vi "Write Ramp Volt.vi"(8 "error in":errorcluster, 10 "Voltage_Ramp":dbl, 11 "89XX in":refnum<class "89XX.lvclass">) -> (0 "error out":errorcluster, 3 "89XX out":refnum<class "89XX.lvclass">)   [LabVIEW 2019, in "89XX.lvlib" / "89XX.lvclass"]
uses:
  Library/89XX.lvclass
  C:/Users/Public/Documents/Development/builds/Engine/Monitored Actor.lvlibp/Monitored Actor/Monitored Actor/Monitored Actor.lvclass
  builds/Engine/Monitored Actor.lvlibp/Monitored Actor/Monitored Actor/Read Actor Label.vi
  builds/Instruments/PowerSupply.lvlibp/Library/PowerSupply.lvclass
  <vilib>/ErrorRing/Error Ring.xnode
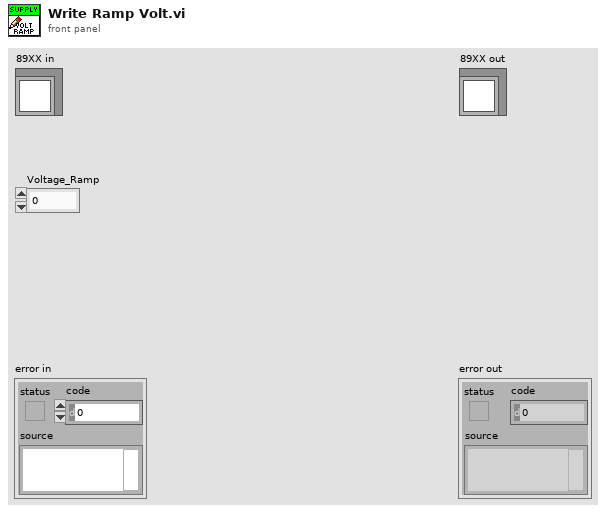
[diagram p1: front panel]
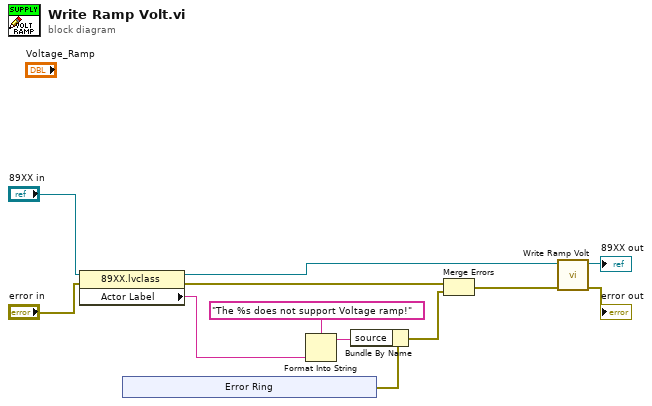
[diagram p0: block diagram]
diagram:
  n1 = property class="89XX.lvclass"(reference="89XX in", error in="error in") -> (reference out=w2:refnum<class "89XX.lvclass">, error out=w10:errorcluster, "Actor Label"=w6:string)
  n2 = xnode "Error Ring"() -> ("error out"=w9:errorcluster)
  n3 = Format Into String(format string="The %s does not support Voltage ramp!", w6) -> (resulting string=w8:string)  [unwired: 2 in, 1 out]
  n4 = Bundle By Name(cluster=w9, "source"=w8) -> (w7:errorcluster)
  n5 = Merge Errors(w10, w7) -> (w1:errorcluster)
  n6 = call-parent "Write Ramp Volt.vi"("error in"=w1, "PowerSupply in"=w2) -> ("error out"=→"error out":errorcluster, "PowerSupply out"=→"89XX out":refnum<class "89XX.lvclass">)  [unwired: 8 in]
